vi "Transmit Command.vi"(4 "Numeric":i64, 6 "String":string, 8 "error in (no error)":errorcluster, 11 "VISA Refnum in":refnum<visa-resource-name>) -> (0 "error out":errorcluster, 2 "read buffer":string, 3 "VISA Refnum out":refnum<visa-resource-name>)   [LabVIEW 2012]
uses:
  <vilib>/Instr/_visa.llb/VISA Flush IO Buffer Mask.ctl
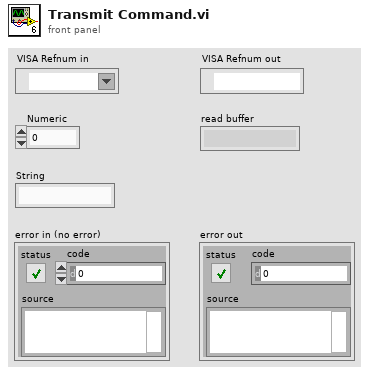
[diagram p1: front panel]
types:
  T1 = typedef "VISA Flush IO Buffer Mask.ctl" = u16
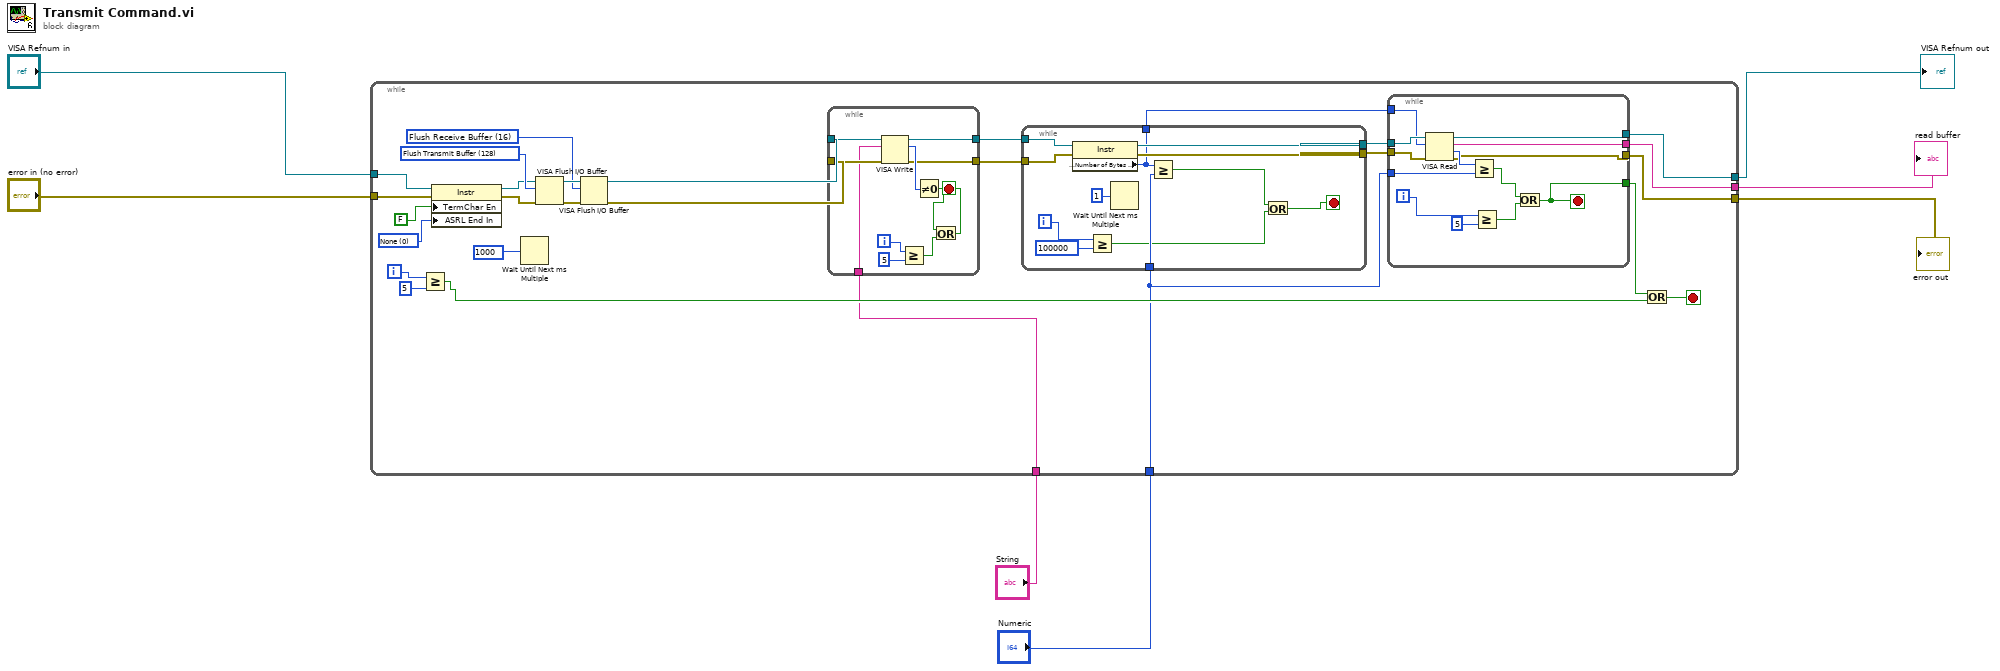
[diagram p0: block diagram]
diagram:
  n1 = while {
    tunnel: "VISA Refnum in" -> [w27]
    tunnel: "error in (no error)" -> [w28]
    tunnel: [w17] -> w7
    tunnel: [w16] -> w5
    tunnel: [w15] -> w6
    tunnel: "String" -> [w9]
    tunnel: "Numeric" -> [w8]
    i -> [w14]
    stop <- w10 stop-if-true
    w29 = u16 0 items=["None", "Last Bit", "TermChar"] ("Serial Settings:End Mode for Reads")
    w32 = T1 16 items=["Flush Receive Buffer"=16, "Write Transmit Buffer to Device"=32, "Flush Receive Buffer (No I/O)"=64, "Flush Transmit Buffer"=128] ("Mask")
    w35 = T1 128 items=["Flush Receive Buffer"=16, "Write Transmit Buffer to Device"=32, "Flush Receive Buffer (No I/O)"=64, "Flush Transmit Buffer"=128] ("Mask")
    n2 = Greater Or Equal?(x=w14, y=5) -> (x >= y?=w11:bool)
    n3 = property class="Instr"(reference=w27, error in=w28, "TermChar En"=FALSE ("Message Based Settings:Termination Character Enable"), "ASRL End In"=w29) -> (reference out=w26:refnum<visa-resource-name>, error out=w25:errorcluster)
    n4 = Wait Until Next ms Multiple(millisecond multiple=u32 1000) -> ()  [unwired: 1 out]
    n5 = VISA Flush I/O Buffer(VISA resource name=w26, mask (16)=w35, error in (no error)=w25) -> (VISA resource name out=w34:refnum<visa-resource-name>, error out=w33:errorcluster)
    n6 = VISA Flush I/O Buffer(VISA resource name=w34, mask (16)=w32, error in (no error)=w33) -> (VISA resource name out=w24:refnum<visa-resource-name>, error out=w23:errorcluster)
    n7 = while {
      tunnel: w24 -> [w71]
      tunnel: w23 -> [w70]
      tunnel: [w68] -> w22
      tunnel: [w67] -> w21
      tunnel: w9 -> [w61]
      i -> [w65]
      stop <- w62 stop-if-true
      n8 = VISA Write(VISA resource name=w71, write buffer=w61, error in (no error)=w70) -> (VISA resource name out=w68:refnum<visa-resource-name>, return count=w69:u32, error out=w67:errorcluster)
      n9 = Greater Or Equal?(x=w65, y=5) -> (x >= y?=w64:bool)
      n10 = Not Equal To 0?(x=w69) -> (x != 0?=w63:bool)
      n11 = Or(x=w63, y=w64) -> (x .or. y?=w62:bool)
    }
    n12 = while {
      tunnel: w22 -> [w60]
      tunnel: w21 -> [w59]
      tunnel: [w58] -> w20
      tunnel: [w57] -> w19
      tunnel: [w55] -> w18
      tunnel: w8 -> [w56]
      i -> [w53]
      stop <- w49 stop-if-true
      n13 = property class="Instr"(reference=w60, error in=w59) -> (reference out=w58:refnum<visa-resource-name>, error out=w57:errorcluster, "Serial Settings:Number of Bytes at Serial Port"=w55:u32)
      n14 = Greater Or Equal?(x=w53, y=100000) -> (x >= y?=w51:bool)
      n15 = Wait Until Next ms Multiple(millisecond multiple=u32 1) -> ()  [unwired: 1 out]
      n16 = Greater Or Equal?(x=w55, y=w56) -> (x >= y?=w50:bool)
      n17 = Or(x=w50, y=w51) -> (x .or. y?=w49:bool)
    }
    n18 = while {
      tunnel: w20 -> [w48]
      tunnel: w19 -> [w47]
      tunnel: w18 -> [w46]
      tunnel: [w44] -> w17
      tunnel: [w36] -> w16
      tunnel: [w37] -> w15
      tunnel: [w39] -> w12
      tunnel: w8 -> [w38]
      i -> [w43]
      stop <- w39 stop-if-true
      n19 = VISA Read(VISA resource name=w48, byte count=w46, error in (no error)=w47) -> (VISA resource name out=w36:refnum<visa-resource-name>, read buffer=w44:string, return count=w45:u32, error out=w37:errorcluster)
      n20 = Greater Or Equal?(x=w45, y=w38) -> (x >= y?=w41:bool)
      n21 = Greater Or Equal?(x=w43, y=5) -> (x >= y?=w40:bool)
      n22 = Or(x=w41, y=w40) -> (x .or. y?=w39:bool)
    }
    n23 = Or(x=w12, y=w11) -> (x .or. y?=w10:bool)
  }
  "read buffer" <- w7
  "error out" <- w6
  "VISA Refnum out" <- w5
